vi "Stepping Example (LabVIEW2014).vi"() -> ()   [LabVIEW 2014]
doc: "This example detects and responds to a service request (SRQ) event. It shows a generic method to generate and handle an SRQ event. But each instrument that supports SRQ event assertion will use a different set of commands than what is shown in this example. You will need to refer to the programmer reference manual for your particular instrument to determine the correct set of commands."
uses:
  <vilib>/regexp/Match Regular Expression.xnode
panel:
  out "die info":string
  out "Home Position":string
  out "Machine":string
  in  "VISA GPIB Resource":refnum<visa-resource-name>="GPIB0::13::INSTR"
  out "Die Info":string
  out "next die":string
  # "SENTIO Remote Control Example - DieStepping"
  # "Query Machine"
  # "Step 1: StepToHome"
  # "Step 4: Get Die Info"
  # "Step 2: Step to First Die"
  # "Step 3: Next Die"
  # "Please setting the wafer map before execute this program"
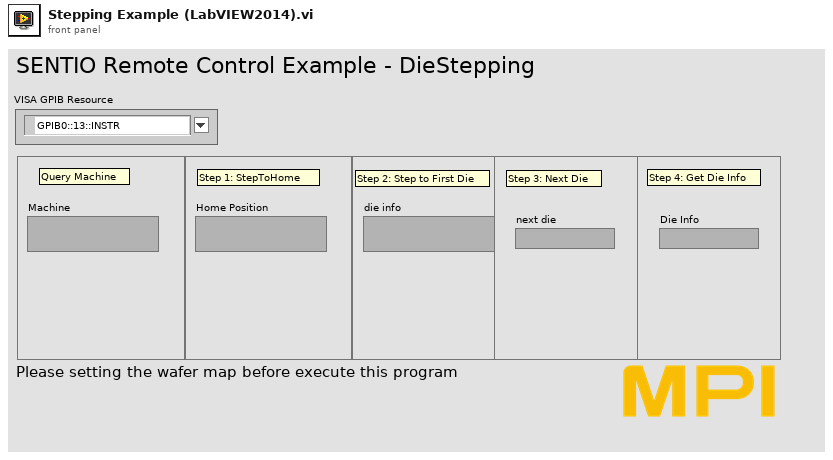
[diagram p1: front panel]
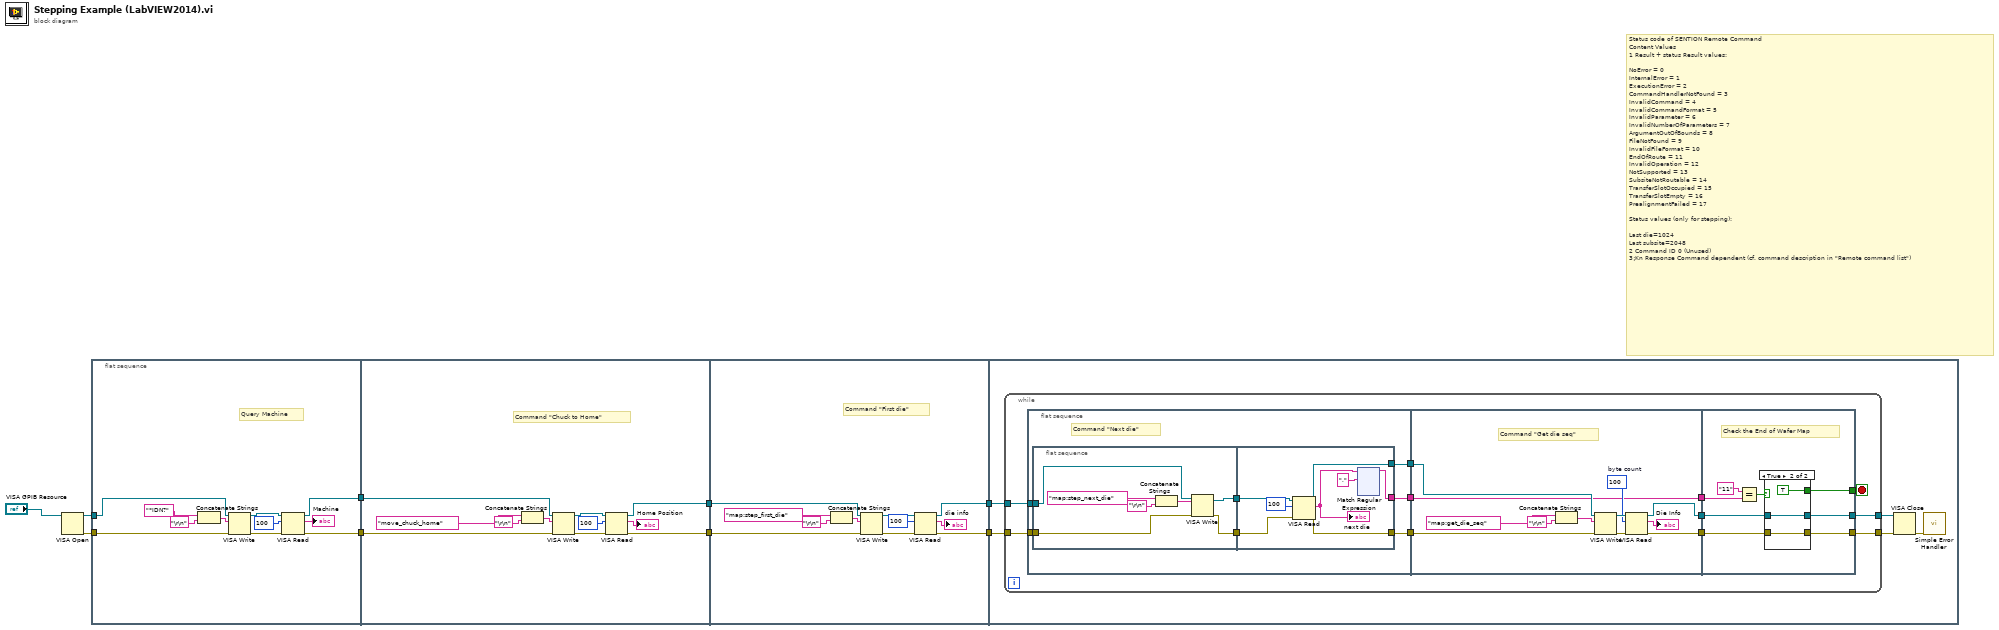
[diagram p0: block diagram]
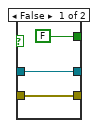
[diagram p2: hidden frame]
diagram:
  # "Status code of SENTION Remote Command \nContent\tValues\n1\tResult + status\tResult values:\n\nNoError = 0\nInternalError = 1\nExecutionError = 2\nCommandHandlerNotFound = 3\nInvalidCommand = 4\nInvalidCommandFormat = 5\nInvalidParameter = 6\nInvalidNumberOfParameters = 7\nArgumentOutOfBounds = 8\nFileNotFound = 9\nInvalidFileFormat = 10\nEndOfRoute = 11\nInvalidOperation = 12\nNotSupported = 13\nSubsiteNotRoutable = 14\nTransferSlotOccupied = 15\nTransferSlotEmpty = 16\nPrealignmentFailed = 17\n\nStatus values (only for stepping):\n\nLast die=1024\nLast subsite=2048\n2\tCommand ID\t0 (Unused)\n3¡Kn\tResponse\tCommand dependent (cf. command description in \"Remote command list\")"
  n1 = VISA Open(VISA resource name="VISA GPIB Resource") -> (VISA resource name=w8:refnum<visa-resource-name>, error out=w7:errorcluster)  [unwired: 1 in, 3 out]
  n2 = flat-sequence {
    tunnel: w8 -> [w20]
    tunnel: w7 -> [w19]
    tunnel: [w14] -> w6
    tunnel: [w13] -> w5
    tunnel: [w22] -> w4
    tunnel: [w21] -> w3
    tunnel: w6 -> [w28]
    tunnel: w5 -> [w27]
    tunnel: w4 -> [w37]
    tunnel: w3 -> [w36]
    tunnel: [w35] -> w2
    tunnel: [w34] -> w1
    tunnel: w2 -> [w46]
    tunnel: w1 -> [w45]
    frame #0 {
      # "Query Machine"
      n3 = Concatenate Strings("*IDN?" ("write buffer"), "\r\n") -> (w10:string)
      n4 = VISA Write(VISA resource name=w20, write buffer=w10, error in (no error)=w19) -> (VISA resource name out=w16:refnum<visa-resource-name>, error out=w15:errorcluster)  [unwired: 1 out]
      n5 = VISA Read(VISA resource name=w16, byte count=u32 100, error in (no error)=w15) -> (VISA resource name out=w14:refnum<visa-resource-name>, read buffer=→"Machine":string, error out=w13:errorcluster)  [unwired: 1 out]
    }
    frame #1 {
      # "Command \"Chuck to Home\""
      n6 = Concatenate Strings("move_chuck_home" ("Command"), "\r\n") -> (w31:string)
      n7 = VISA Write(VISA resource name=w28, write buffer=w31, error in (no error)=w27) -> (VISA resource name out=w24:refnum<visa-resource-name>, error out=w23:errorcluster)  [unwired: 1 out]
      n8 = VISA Read(VISA resource name=w24, byte count=u32 100, error in (no error)=w23) -> (VISA resource name out=w22:refnum<visa-resource-name>, read buffer=→"Home Position":string, error out=w21:errorcluster)  [unwired: 1 out]
    }
    frame #2 {
      # "Command \"First die\""
      n9 = Concatenate Strings("map:step_first_die" ("Command"), "\r\n") -> (w38:string)
      n10 = VISA Write(VISA resource name=w37, write buffer=w38, error in (no error)=w36) -> (VISA resource name out=w33:refnum<visa-resource-name>, error out=w42:errorcluster)  [unwired: 1 out]
      n11 = VISA Read(VISA resource name=w33, byte count=u32 100, error in (no error)=w42) -> (VISA resource name out=w35:refnum<visa-resource-name>, read buffer=→"die info":string, error out=w34:errorcluster)  [unwired: 1 out]
    }
    frame #3 {
      n12 = while {
        tunnel: w46 -> [w56]
        tunnel: w45 -> [w55]
        tunnel: [w52] -> w44
        tunnel: [w50] -> w43
        stop <- w53 stop-if-true
        n13 = flat-sequence {
          tunnel: [w65] -> w58
          tunnel: [w64] -> w57
          tunnel: w56 -> [w63]
          tunnel: w55 -> [w62]
          tunnel: [w60] -> w48
          tunnel: w58 -> [w203]
          tunnel: w57 -> [w202]
          tunnel: [w195] -> w54
          tunnel: [w197] -> w51
          tunnel: [w196] -> w49
          tunnel: w48 -> [w195]
          tunnel: w54 -> [w212]
          tunnel: [w211] -> w53
          tunnel: [w210] -> w52
          tunnel: w51 -> [w209]
          tunnel: [w208] -> w50
          tunnel: w49 -> [w207]
          frame #0 {
            # "Command \"Next die\""
            n14 = flat-sequence {
              tunnel: [w66] -> w61
              tunnel: w63 -> [w69]
              tunnel: w62 -> [w67]
              tunnel: [w68] -> w59
              tunnel: w61 -> [w74]
              tunnel: [w75] -> w65
              tunnel: [w73] -> w64
              tunnel: [w79] -> w60
              tunnel: w59 -> [w77]
              frame #0 {
                n15 = Concatenate Strings("map:step_next_die" ("Command"), "\r\n") -> (w70:string)
                n16 = VISA Write(VISA resource name=w69, write buffer=w70, error in (no error)=w67) -> (VISA resource name out=w68:refnum<visa-resource-name>, error out=w66:errorcluster)  [unwired: 1 out]
              }
              frame #1 {
                n17 = VISA Read(VISA resource name=w77, byte count=100, error in (no error)=w74) -> (VISA resource name out=w75:refnum<visa-resource-name>, read buffer=w76:string, error out=w73:errorcluster)  [unwired: 1 out]
                "next die" <- w76
                n18 = xnode "Match Regular Expression"("input string"=w76, "regular expression"=",") -> ("before match"=w79:string)  [unwired: 4 in, 4 out]
              }
            }
          }
          frame #1 {
            w198 = u32 100  # byte count
            # "Command \"Get die seq\""
            n19 = Concatenate Strings("map:get_die_seq" ("Command"), "\r\n") -> (w204:string)
            n20 = VISA Write(VISA resource name=w203, write buffer=w204, error in (no error)=w202) -> (VISA resource name out=w199:refnum<visa-resource-name>, error out=w200:errorcluster)  [unwired: 1 out]
            n21 = VISA Read(VISA resource name=w199, byte count=w198, error in (no error)=w200) -> (VISA resource name out=w197:refnum<visa-resource-name>, read buffer=→"Die Info":string, error out=w196:errorcluster)  [unwired: 1 out]
          }
          frame #2 {
            # "Check the End of Wafer Map"
            n22 = Equal?(x="11", y=w212) -> (x = y?=w214:bool)
            n23 = case shown="True" w214 {
              tunnel: [FALSE TRUE] -> w211
              tunnel: [w216 w219] -> w210
              tunnel: w209 -> [w216 w219]
              tunnel: [w215 w218] -> w208
              tunnel: w207 -> [w215 w218]
              frame False {
              }
              frame True {
              }
            }
          }
        }
      }
      n24 = VISA Close(VISA resource name=w44, error in (no error)=w43) -> (error out=w47:errorcluster)
      n25 = call <vilib>:"Simple Error Handler.vi"("error in (no error)"=w47) -> ()  [unwired: 1 in, 8 out]
    }
  }
